vi "GetDebugInfoString.vi"(11 "CDependencyList in":refnum<class "CDependencyList.lvclass">) -> (1 "Debug info":string, 3 "CDependencyList":refnum<class "CDependencyList.lvclass">)   [LabVIEW 2020, in "DependencyInspection.lvlib" / "CDependencyList.lvclass"]
uses:
  CDependencyList.lvclass
  LabVIEWObjectInterfaces/ILabVIEWItem/ILabVIEWItem.lvclass
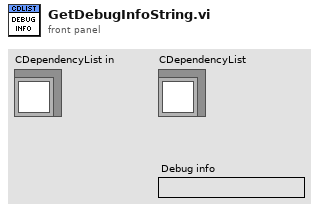
[diagram p1: front panel]
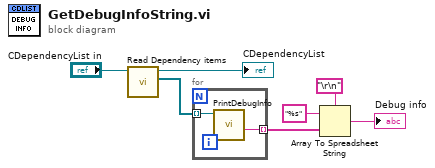
[diagram p0: block diagram]
diagram:
  n1 = call-dynamic "Read Dependency items.vi"("CDependencyList in"="CDependencyList in") -> ("Dependency items"=w5:refnum<class "ILabVIEWItem.lvclass">[], "CDependencyList out"=→"CDependencyList":refnum<class "CDependencyList.lvclass">)  [unwired: 9 in]
  n2 = for {
    tunnel: w5 -> [w9] mode=indexing
    tunnel: [w8] -> w2 mode=indexing
    n3 = call-dynamic "PrintDebugInfo.vi"("ILabVIEWItem in"=w9) -> ("Debug string"=w8:string)  [unwired: 8 in, 2 out]
  }
  n4 = Array To Spreadsheet String(delimiter (Tab)="\r\n", array=w2, 3:"%s" ("format string")) -> (spreadsheet string=→"Debug info":string)
